vi "read_raw_dataV3.0.vi"() -> ()   [LabVIEW 2017]
uses:
  <vilib>/Utility/file.llb/Read Delimited Spreadsheet (I64).vi
  <vilib>/Utility/file.llb/Write Delimited Spreadsheet (string).vi
  <vilib>/Utility/file.llb/Write Delimited Spreadsheet (DBL).vi
  <vilib>/Utility/file.llb/Write Delimited Spreadsheet (I64).vi
panel:
  out "element":ext
  out "appended array":dbl[](array[numeric])=[965934467999.937, 965934467999.922] format="%.00000f"
  out "x .and. y?":u64=28
  out "time 2":dbl=965934466000.0 format="%.000f"
  out "x*y":dbl=0.078
  out "x-y":dbl=1999.922
  out "x+y":u32=39
  in  "col":i32
  in  "file path (dialog if empty)":path=path "G:/tdc/2017/code_density_rom.mem"
  out "size(s)":i32[](array[numeric])=[2048, 128]
  out "Array":u32[][](array[numeric]) format="%x"
  out "cal":u32[][](graph)
  out "x/y":dbl=0.002
  out "index":i32=1
  out "time":dbl=965934467999.922 format="%.00000f"
  in  "通道数量":i32=128
  out "fine":u64=737 format="%x"
  out "data 5":string
  in  "ch list":u16[](array[numeric])=[0, 1, 2, 3, 4, 5, 6, 7]
  in  "codeDensity":path=path "G:/tdc/2017/data/112_codedesity.csv"
  out "file path (dialog if empty) 2":path=path "G:/tdc/2017/test_20240327_022214.txt"
  out "ip":u64 format="%x"
  out "data 9":string
  out "result string":string="test_20250325_114227"
  out "sent number":u64=7168 format="%x"
  out "trigger number":u64=42496 format="%x"
  out "data 8":string
  out "data 7":string
  out "data":u64[](array[numeric])=[35, 5, 71, 71, 31675062850000] format="%x"
  out "data 2":string
  out "data 4":string
  out "coarse time":u64=482967233 format="%x"
  out "error out":errorcluster
  out "substring":string
  out "number 3":u32
  out "channel number":u64=28 format="%x"
  in  "channel":u64
  out "data 3":string="Z"
  in  "dat file (use dialog)":path=path "G:/tdc/2017/test_20250325_114227.dat"
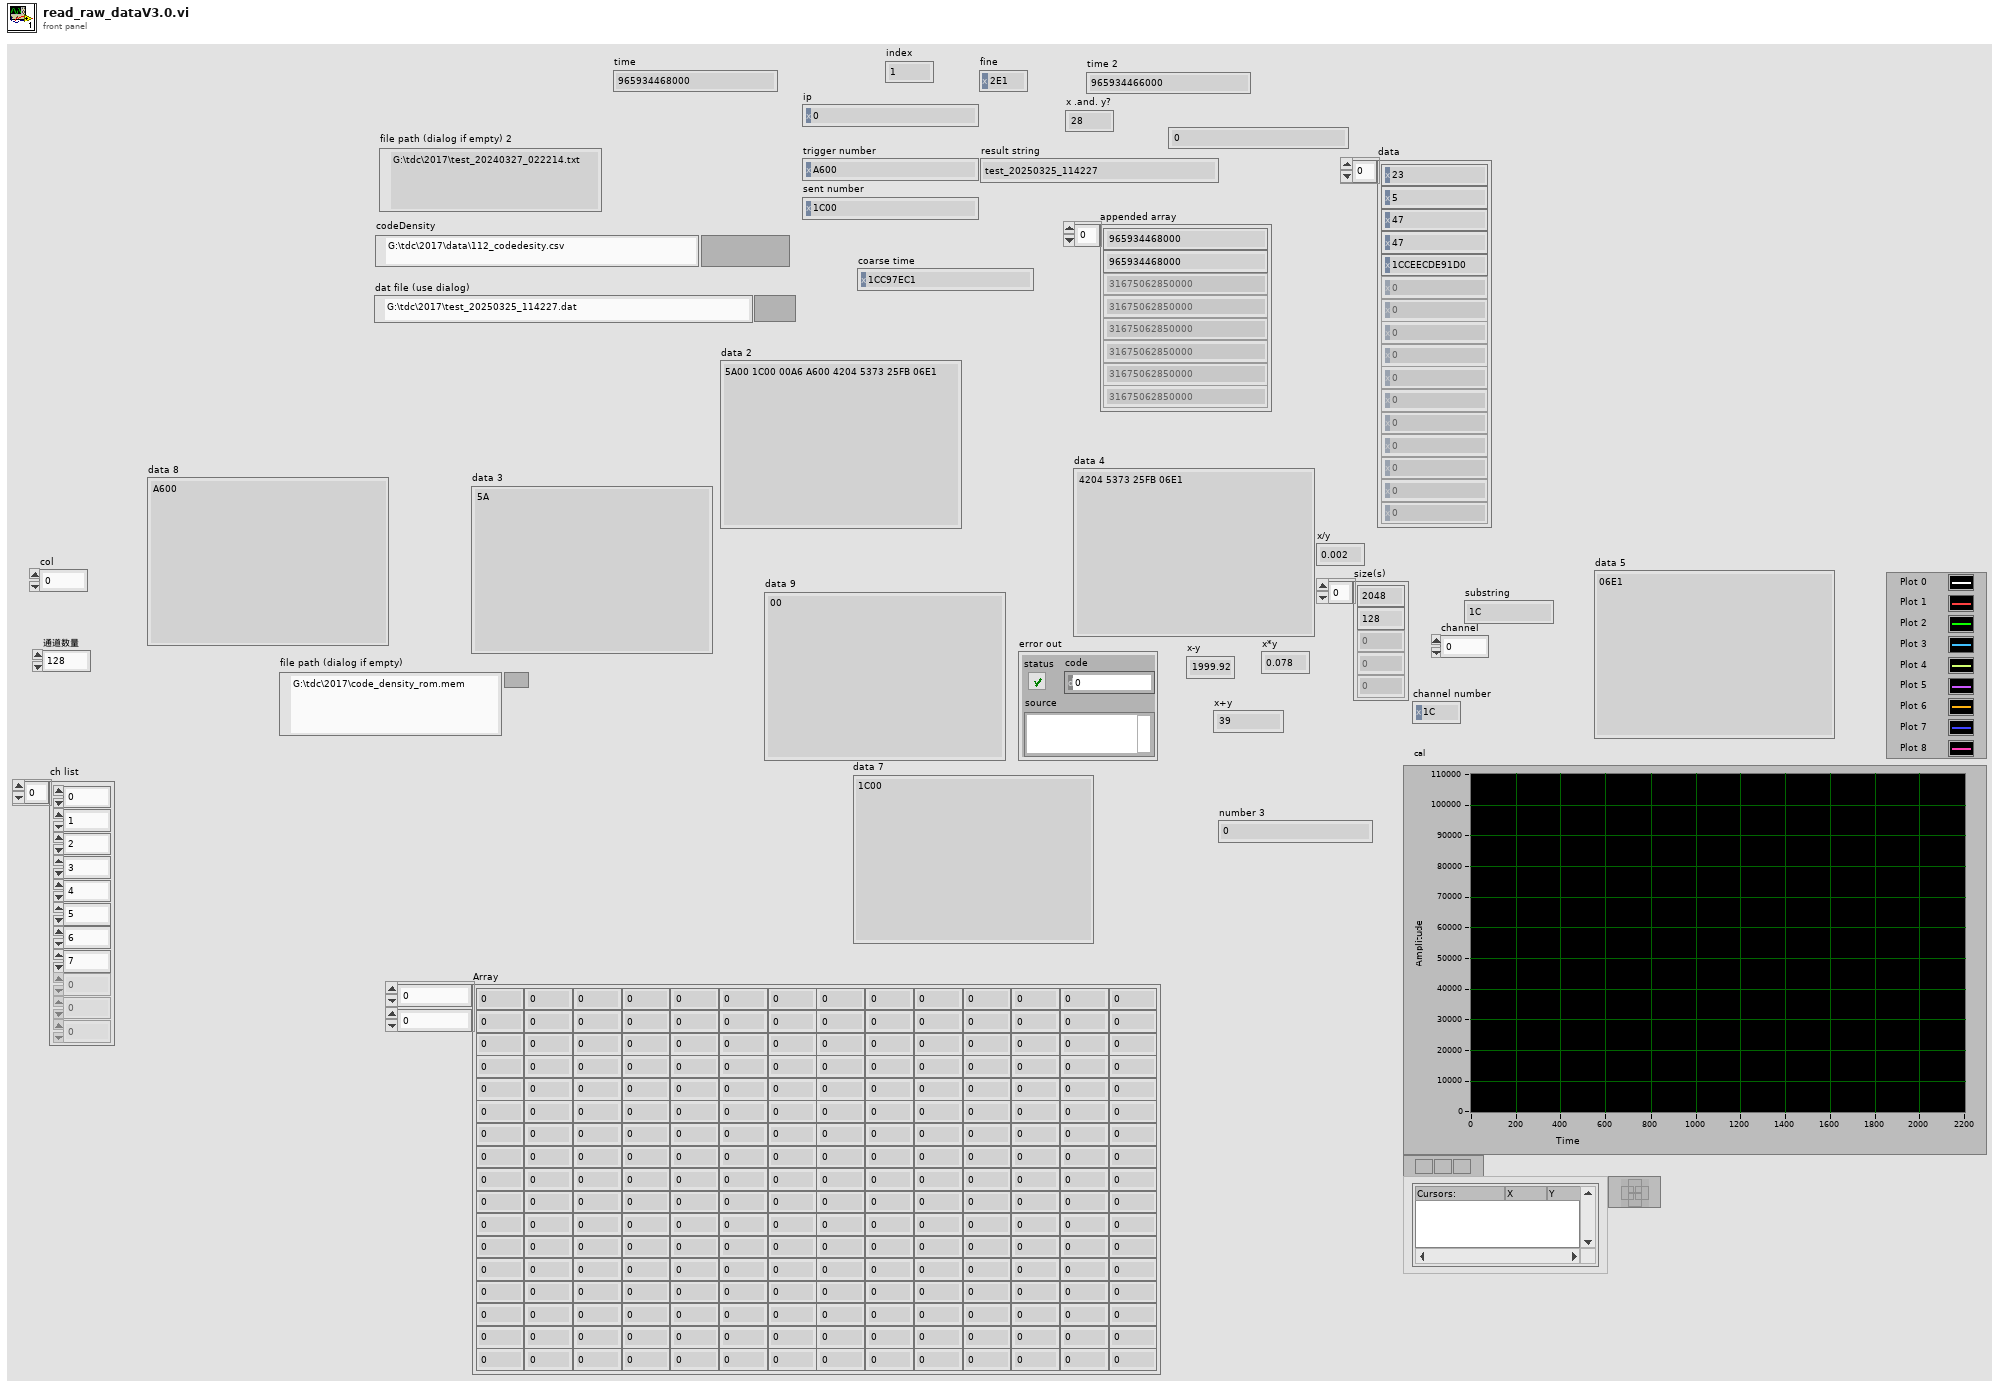
[diagram p1: front panel]
types:
  T1 = enum16{"open", "replace", "create", "open or create", "replace or create", "replace or create with confirmation"}
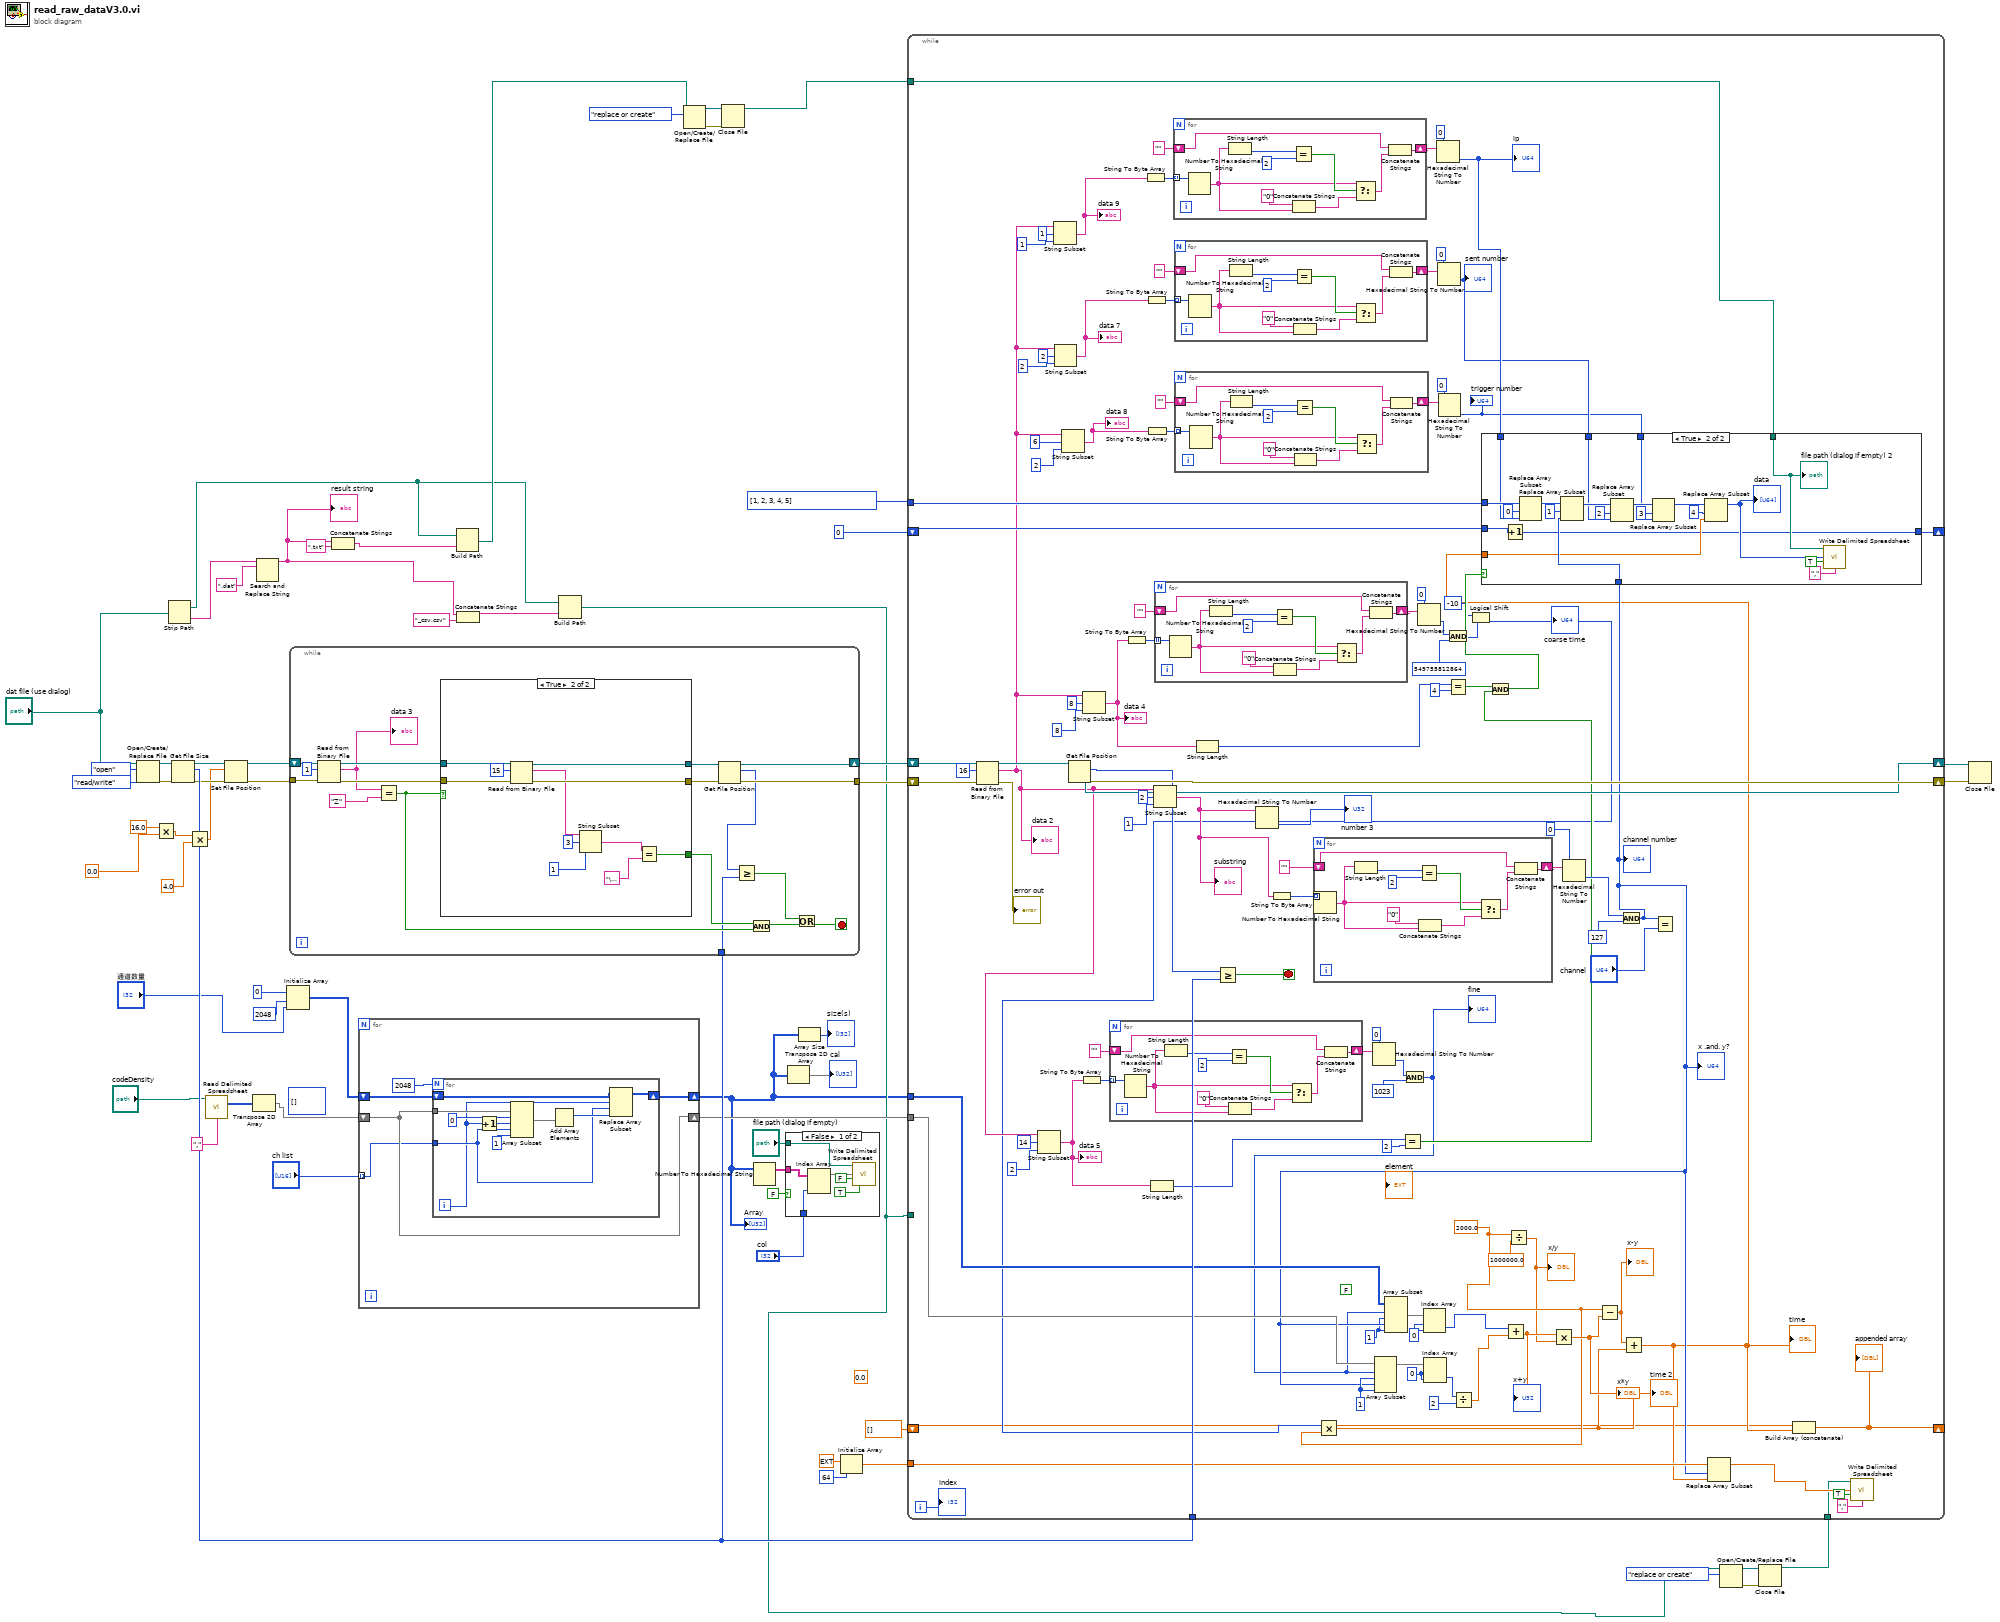
[diagram p0: block diagram]
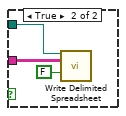
[diagram p2: hidden frame]
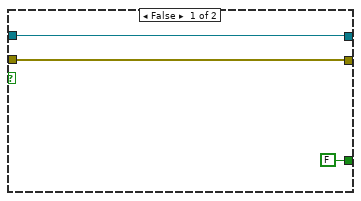
[diagram p4: hidden frame]
diagram:
  (unwired) 0.0
  (unwired) i64[][] []
  n1 = Open/Create/Replace File(file path (use dialog)="dat file (use dialog)", operation (0:open)=T1."open", access (0:read/write)=enum16{"read/write", "read-only", "write-only"}."read/write") -> (refnum out=w60:refnum<file>, error out=w55:errorcluster)  [unwired: 3 in, 1 out]
  n2 = Multiply(x=16.0, y=0.0) -> (x*y=w21:dbl)
  n3 = Strip Path(path="dat file (use dialog)") -> (stripped path=w10:path, name=w48:string)
  n4 = Get File Size(file=w60, error in=w55) -> (refnum out=w27:refnum<file>, size (in bytes)=w50:i64, 0:w25:errorcluster)
  n5 = Multiply(x=w21, y=4.0) -> (x*y=w19:dbl)
  n6 = call-poly <vilib>:"Read Delimited Spreadsheet.vi"("file path (dialog if empty)"="codeDensity", "delimiter (\\t)"="," ("delimiter (\\t)")) -> ("all rows"=w44:i64[][])  [unwired: 8 in, 5 out]
  n7 = Set File Position(offset (in bytes) (0)=w19, refnum=w27, error in=w25) -> (refnum out=w26:refnum<file>, error out=w24:errorcluster)  [unwired: 1 in]
  n8 = Transpose 2D Array(2D array=w44) -> (transposed array=w32:i64[][])
  n9 = Search and Replace String(input string=w48, search string=".dat") -> (result string=w12:string)  [unwired: 6 in, 3 out]
  "result string" <- w12
  n10 = Initialize Array(u32 0 ("element"), 2048 ("dimension size"), "通道数量") -> (w33:u32[][])
  n11 = while {
    tunnel: w24 -> [w77]
    shift-right: [w65] -> w56
    shift-left: w26 -> [w78]
    tunnel: [w66] -> w57
    tunnel: w50 -> [w64]
    stop <- w62 stop-if-true
    n12 = Read from Binary File(8:w77, 10:1 ("count (1)"), 11:w78) -> (0:w73:errorcluster, 2:w71:string, 3:w74:refnum<file>)  [unwired: 3 in, 1 out]
    "data 3" <- w71
    n13 = Equal?(x=w71, y="Z") -> (x = y?=w68:bool)
    n14 = case shown="True" w68 {
      tunnel: w74 -> [w81 w92]
      tunnel: w73 -> [w80 w91]
      tunnel: [w81 w89] -> w72
      tunnel: [w80 w88] -> w67
      tunnel: [FALSE w82] -> w69
      frame False {
      }
      frame True {
        n15 = Read from Binary File(8:w91, 10:15 ("count (1)"), 11:w92) -> (0:w88:errorcluster, 2:w85:string, 3:w89:refnum<file>)  [unwired: 3 in, 1 out]
        n16 = String Subset(string=w85, offset (0)=3, length (rest)=1 ("length (rest)")) -> (substring=w84:string)
        n17 = Equal?(x=w84, y="\u0000") -> (x = y?=w82:bool)
      }
    }
    n18 = Get File Position(4:w67, 7:w72) -> (0:w66:errorcluster, 2:w63:i64, 3:w65:refnum<file>)
    n19 = Greater Or Equal?(x=w63, y=w64) -> (x >= y?=w61:bool)
    n20 = Compound Arithmetic op=AND(w69, w68) -> (w70:bool)
    n21 = Or(x=w61, y=w70) -> (x .or. y?=w62:bool)
  }
  n22 = Concatenate Strings(w12, ".txt" ("string")) -> (w45:string)
  n23 = for {
    shift-right: [w95] -> w5
    shift-left: w33 -> [w96]
    shift-right: [w94] -> w40
    shift-left: w32 -> [w94]
    tunnel: "ch list" -> [w93] mode=indexing
    n24 = for {
      N: 2048 -> [_]
      tunnel: w94 -> [w107]
      tunnel: w93 -> [w100]
      shift-right: [w102] -> w95
      shift-left: w96 -> [w103]
      i -> [w99]
      n25 = Increment(x=w99) -> (x+1=w98:i32)
      n26 = Array Subset(array=w107, index (row)=0 ("索引"), length (row)=w98, index (col)=w100, length (col)=1 ("长度")) -> (w104:i64[][])
      n27 = Add Array Elements(numeric array=w104) -> (sum=w101:i64)
      n28 = Replace Array Subset(array=w103, new element=w101, index (row)=w99, index (col)=w100) -> (w102:u32[][])
    }
  }
  "Array" <- w5
  n29 = Build Path(base path=w10, name or relative path=w45) -> (appended path=w15:path)
  n30 = Concatenate Strings(w12, "_csv.csv" ("string")) -> (w11:string)
  n31 = Build Path(base path=w10, name or relative path=w11) -> (appended path=w9:path)
  n32 = Open/Create/Replace File(file path (use dialog)=w15, operation (0:open)=T1."replace or create") -> (refnum out=w16:refnum<file>, error out=w17:errorcluster)  [unwired: 4 in, 1 out]
  n33 = Close File(refnum=w16, error in=w17) -> (path=w14:path)  [unwired: 1 out]
  n34 = Number To Hexadecimal String(2:w5) -> (0:w4:string[][])  [unwired: 1 in]
  n35 = case shown="False" FALSE {
    tunnel: "file path (dialog if empty)" -> [w112 w116]
    tunnel: w4 -> [w111 w114]
    tunnel: "col" -> [w109 _]
    frame False {
      n36 = Index Array(array=w111, index (col)=w109) -> (element=w110:string[])  [unwired: 1 in]
      n37 = call-poly <vilib>:"Write Delimited Spreadsheet.vi"("file path (dialog if empty)"=w112, "1D data"=w110, "append to file? (new file:F)"=FALSE, "transpose? (no:F)"=TRUE) -> ()  [unwired: 10 in, 2 out]
    }
    frame True {
      n38 = call-poly <vilib>:"Write Delimited Spreadsheet.vi"("file path (dialog if empty)"=w116, "2D data"=w114, "append to file? (new file:F)"=FALSE) -> ()  [unwired: 11 in, 2 out]
    }
  }
  n39 = Transpose 2D Array(2D array=w5) -> (transposed array=→"cal":u32[][])
  n40 = Array Size(array=w5) -> (size(s)=→"size(s)":i32[])
  n41 = Initialize Array(ext 0.0 ("element"), 64 ("dimension size")) -> (w37:ext[])
  n42 = Open/Create/Replace File(file path (use dialog)=w9, operation (0:open)=T1."replace or create") -> (refnum out=w29:refnum<file>, error out=w30:errorcluster)  [unwired: 4 in, 1 out]
  n43 = Close File(refnum=w29, error in=w30) -> (path=w28:path)  [unwired: 1 out]
  n44 = while {
    shift-right: [w219] -> w54
    shift-left: w56 -> [w223]
    shift-right: [w221] -> w53
    shift-left: w57 -> [w224]
    tunnel: w50 -> [w217]
    shift-right: [w165] -> _
    shift-left: 0 ("length (rest)") -> [w196]
    tunnel: w14 -> [w166]
    tunnel: u64[] [1, 2, 3, 4, 5] -> [w195]
    tunnel: w5 -> [w141]
    tunnel: w40 -> [w142]
    tunnel: w37 -> [w138]
    tunnel: w28 -> [w131]
    tunnel: w9 -> [_]
    shift-right: [w119] -> _
    shift-left: dbl[] [] -> [w117]
    i -> [w130]
    stop <- w216 stop-if-true
    w132 = 0 ("index (row)")
    w134 = 1 ("长度")
    w144 = 2000.0 ("x")
    (unwired) FALSE
    w157 = 0 ("索引 (行)")
    w159 = 1 ("长度")
    n45 = Read from Binary File(8:w224, 10:16 ("count (1)"), 11:w223) -> (0:→"error out":errorcluster, 2:w145:string, 3:w220:refnum<file>)  [unwired: 3 in, 1 out]
    "data 2" <- w145
    n46 = String Subset(string=w145, offset (0)=14, length (rest)=2 ("length (rest)")) -> (substring=w148:string)
    "data 5" <- w148
    n47 = String Subset(string=w145, offset (0)=1, length (rest)=1 ("length (rest)")) -> (substring=w176:string)
    "data 9" <- w176
    n48 = String Subset(string=w145, offset (0)=2, length (rest)=2 ("length (rest)")) -> (substring=w177:string)
    "data 7" <- w177
    n49 = String Subset(string=w145, offset (0)=6, length (rest)=2 ("length (rest)")) -> (substring=w182:string)
    "data 8" <- w182
    n50 = Get File Position(7:w220) -> (0:w221:errorcluster, 2:w218:i64, 3:w219:refnum<file>)  [unwired: 1 in]
    n51 = String To Byte Array(string=w148) -> (unsigned byte array=w151:u8[])
    n52 = String Subset(string=w145, offset (0)=8, length (rest)=8 ("length (rest)")) -> (substring=w193:string)
    "data 4" <- w193
    n53 = for {
      shift-right: [w233] -> w150
      shift-left: "" ("format string") -> [w230]
      tunnel: w151 -> [w234] mode=indexing
      n54 = Number To Hexadecimal String(2:w234) -> (0:w226:string)  [unwired: 1 in]
      n55 = String Length(string=w226) -> (length=w232:i32)
      n56 = Equal?(x=w232, y=2) -> (x = y?=w229:bool)
      n57 = Concatenate Strings("0" ("format string"), w226) -> (w228:string)
      n58 = Select(t=w226, s=w229, f=w228) -> (s? t:f=w225:string)
      n59 = Concatenate Strings(w230, w225) -> (w233:string)
    }
    n60 = String To Byte Array(string=w193) -> (unsigned byte array=w212:u8[])
    n61 = String To Byte Array(string=w176) -> (unsigned byte array=w173:u8[])
    n62 = String To Byte Array(string=w177) -> (unsigned byte array=w180:u8[])
    n63 = String To Byte Array(string=w182) -> (unsigned byte array=w184:u8[])
    n64 = String Length(string=w148) -> (length=w147:i32)
    n65 = String Subset(string=w145, offset (0)=2, length (rest)=1 ("length (rest)")) -> (substring=w199:string)
    "substring" <- w199
    n66 = for {
      shift-right: [w305] -> w211
      shift-left: "" ("format string") -> [w302]
      tunnel: w212 -> [w306] mode=indexing
      n67 = Number To Hexadecimal String(2:w306) -> (0:w298:string)  [unwired: 1 in]
      n68 = String Length(string=w298) -> (length=w304:i32)
      n69 = Equal?(x=w304, y=2) -> (x = y?=w301:bool)
      n70 = Concatenate Strings("0" ("format string"), w298) -> (w300:string)
      n71 = Select(t=w298, s=w301, f=w300) -> (s? t:f=w297:string)
      n72 = Concatenate Strings(w302, w297) -> (w305:string)
    }
    n73 = for {
      shift-right: [w243] -> w174
      shift-left: "" ("format string") -> [w240]
      tunnel: w173 -> [w244] mode=indexing
      n74 = Number To Hexadecimal String(2:w244) -> (0:w236:string)  [unwired: 1 in]
      n75 = String Length(string=w236) -> (length=w242:i32)
      n76 = Equal?(x=w242, y=2) -> (x = y?=w239:bool)
      n77 = Concatenate Strings("0" ("format string"), w236) -> (w238:string)
      n78 = Select(t=w236, s=w239, f=w238) -> (s? t:f=w235:string)
      n79 = Concatenate Strings(w240, w235) -> (w243:string)
    }
    n80 = for {
      shift-right: [w253] -> w179
      shift-left: "" ("format string") -> [w250]
      tunnel: w180 -> [w254] mode=indexing
      n81 = Number To Hexadecimal String(2:w254) -> (0:w246:string)  [unwired: 1 in]
      n82 = String Length(string=w246) -> (length=w252:i32)
      n83 = Equal?(x=w252, y=2) -> (x = y?=w249:bool)
      n84 = Concatenate Strings("0" ("format string"), w246) -> (w248:string)
      n85 = Select(t=w246, s=w249, f=w248) -> (s? t:f=w245:string)
      n86 = Concatenate Strings(w250, w245) -> (w253:string)
    }
    n87 = for {
      shift-right: [w263] -> w185
      shift-left: "" ("format string") -> [w260]
      tunnel: w184 -> [w264] mode=indexing
      n88 = Number To Hexadecimal String(2:w264) -> (0:w256:string)  [unwired: 1 in]
      n89 = String Length(string=w256) -> (length=w262:i32)
      n90 = Equal?(x=w262, y=2) -> (x = y?=w259:bool)
      n91 = Concatenate Strings("0" ("format string"), w256) -> (w258:string)
      n92 = Select(t=w256, s=w259, f=w258) -> (s? t:f=w255:string)
      n93 = Concatenate Strings(w260, w255) -> (w263:string)
    }
    n94 = String Length(string=w193) -> (length=w191:i32)
    n95 = Greater Or Equal?(x=w218, y=w217) -> (x >= y?=w216:bool)
    n96 = Hexadecimal String To Number(string=w199) -> (number=→"number 3":u32)  [unwired: 2 in, 1 out]
    n97 = String To Byte Array(string=w199) -> (unsigned byte array=w202:u8[])
    n98 = for {
      shift-right: [w295] -> w201
      shift-left: "" ("format string") -> [w292]
      tunnel: w202 -> [w296] mode=indexing
      n99 = Number To Hexadecimal String(2:w296) -> (0:w288:string)  [unwired: 1 in]
      n100 = String Length(string=w288) -> (length=w294:i32)
      n101 = Equal?(x=w294, y=2) -> (x = y?=w291:bool)
      n102 = Concatenate Strings("0" ("format string"), w288) -> (w290:string)
      n103 = Select(t=w288, s=w291, f=w290) -> (s? t:f=w287:string)
      n104 = Concatenate Strings(w292, w287) -> (w295:string)
    }
    n105 = Hexadecimal String To Number(string=w150, default (0uL)=u64 0 ("default (0 U32)")) -> (number=w127:u64)  [unwired: 1 in, 1 out]
    n106 = Equal?(x=w147, y=2) -> (x = y?=w140:bool)
    n107 = And(x=w127, y=u64 1023 ("default (0 U32)")) -> (x .and. y?=w126:u64)
    "fine" <- w126
    n108 = Hexadecimal String To Number(string=w211, default (0uL)=u64 0 ("default (0 U32)")) -> (number=w123:u64)  [unwired: 1 in, 1 out]
    n109 = Hexadecimal String To Number(string=w174, default (0uL)=u64 0 ("default (0 U32)")) -> (number=w169:u64)  [unwired: 1 in, 1 out]
    "ip" <- w169
    n110 = Hexadecimal String To Number(string=w179, default (0uL)=u64 0 ("default (0 U32)")) -> (number=w168:u64)  [unwired: 1 in, 1 out]
    "sent number" <- w168
    n111 = Hexadecimal String To Number(string=w185, default (0uL)=u64 0 ("default (0 U32)")) -> (number=w167:u64)  [unwired: 1 in, 1 out]
    "trigger number" <- w167
    n112 = And(x=w123, y=u64 549755812864 ("port")) -> (x .and. y?=w122:u64)
    n113 = Equal?(x=w191, y=4) -> (x = y?=w192:bool)
    n114 = Logical Shift(y=i16 -10, x=w122) -> (x << y=w129:u64)
    "coarse time" <- w129
    n115 = Multiply(x=w129, y=w144) -> (x*y=w120:dbl)
    "time 2" <- w120
    n116 = And(x=w192, y=w140) -> (x .and. y?=w189:bool)
    n117 = Divide(x=w144, y=1000000.0) -> (x/y=w143:dbl)
    "x/y" <- w143
    n118 = Hexadecimal String To Number(string=w201, default (0uL)=u64 0 ("default (0 U32)")) -> (number=w198:u64)  [unwired: 1 in, 1 out]
    n119 = And(x=w198, y=u64 127 ("default (0 U32)")) -> (x .and. y?=w137:u64)
    "channel number" <- w137
    "x .and. y?" <- w137
    n120 = Array Subset(array=w142, index (row)=w126, length (row)=w159, index (col)=w137, length (col)=w159) -> (w158:i64[][])
    n121 = Array Subset(array=w141, index (row)=w126, length (row)=w134, index (col)=w137, length (col)=w134) -> (w133:u32[][])
    n122 = Index Array(array=w133, index (row)=w132, index (col)=w132) -> (element=w162:u32)
    n123 = Index Array(array=w158, index (row)=w157, index (col)=w157) -> (element=w156:i64)
    n124 = Divide(x=w156, y=u32 2) -> (x/y=w160:dbl)
    n125 = Add(x=w162, y=w160) -> (x+y=w161:dbl)
    "x+y" <- w161
    n126 = Multiply(x=w161, y=w143) -> (x*y=w155:dbl)
    "x*y" <- w155
    n127 = Subtract(x=w144, y=w155) -> (x-y=w124:dbl)
    "x-y" <- w124
    n128 = Add(x=w124, y=w120) -> (x+y=w118:dbl)
    "time" <- w118
    n129 = case shown="True" w189 {
      tunnel: w196 -> [w265 w268]
      tunnel: w195 -> [_ w286]
      tunnel: w118 -> [_ w269]
      tunnel: w169 -> [_ w284]
      tunnel: w168 -> [_ w276]
      tunnel: w167 -> [_ w277]
      tunnel: w137 -> [_ w275]
      tunnel: w166 -> [_ w273]
      tunnel: [w265 w267] -> w165
      frame False {
      }
      frame True {
        n130 = Increment(x=w268) -> (x+1=w267:i32)
        n131 = Replace Array Subset(array=w286, new element=w284, index=0) -> (w283:u64[])
        n132 = Replace Array Subset(array=w283, new element=w275, index=1) -> (w278:u64[])
        n133 = Replace Array Subset(array=w278, new element=w276, index=2) -> (w280:u64[])
        n134 = Replace Array Subset(array=w280, new element=w277, index=3) -> (w271:u64[])
        n135 = Replace Array Subset(array=w271, new element=w269, index=4) -> (w270:u64[])
        "data" <- w270
        n136 = call-poly <vilib>:"Write Delimited Spreadsheet.vi"("file path (dialog if empty)"=w273, "1D data"=w270, "append to file? (new file:F)"=TRUE, "delimiter (\\t)"="," ("delimiter (\\t)")) -> ()  [unwired: 10 in, 2 out]
        "file path (dialog if empty) 2" <- w273
      }
    }
    n137 = Equal?(x=w137, y="channel") -> ()  [unwired: 1 out]
    n138 = Replace Array Subset(array=w138, new element=w118, index=w137) -> (w136:ext[])
    n139 = Build Array (concatenate)(w117, w118) -> (w119:dbl[])
    "appended array" <- w119
    n140 = call-poly <vilib>:"Write Delimited Spreadsheet.vi"("file path (dialog if empty)"=w131, "1D data"=w136, "append to file? (new file:F)"=TRUE, "delimiter (\\t)"="," ("delimiter (\\t)")) -> ()  [unwired: 10 in, 2 out]
    "index" <- w130
  }
  n141 = Close File(refnum=w54, error in=w53) -> ()  [unwired: 2 out]
